vi "WriteOctToFile.vi"(8 "Error In":errorcluster, 9 "Scan.lvclass":refnum<class "Scan.lvclass">, 10 "Refnum in":refnum<file>, 11 "Queue in":refnum<queue>) -> (0 "error out":errorcluster, 1 "refnum out":refnum<file>, 2 "Frame number":dbl, 3 "prepend array or string size? (T)":bool)   [LabVIEW 2017]
uses:
  classes/Scans/Scan.lvclass
  classes/Scans/Scan.lvclass/Scan.ctl
  classes/Scans/Read B scans.vi
  classes/Scans/Read Repeat B scans.vi
  classes/Scans/Read C scans.vi
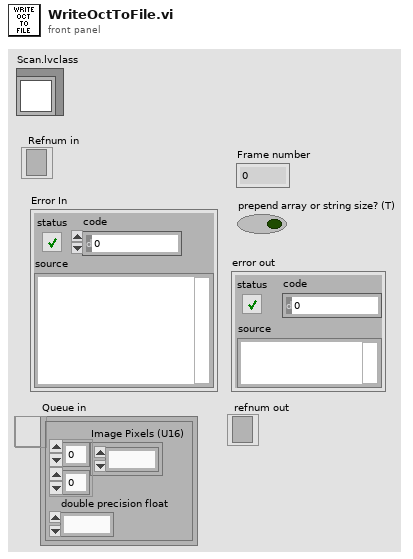
[diagram p1: front panel]
types:
  T1 = enum16{"big-endian, network order", "native, host order", "little-endian"}
  T2 = cluster{"Image Pixels (U16)":u16[][], "double precision float":dbl}
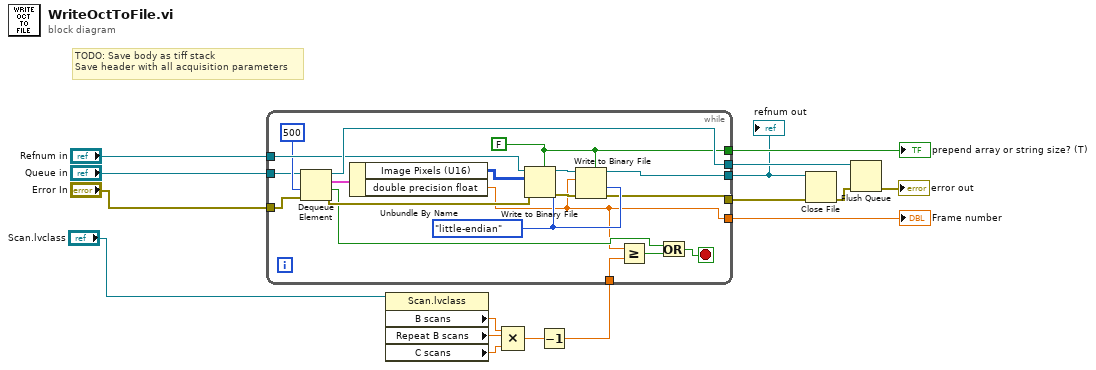
[diagram p0: block diagram]
diagram:
  # "TODO: Save body as tiff stack\nSave header with all acquisition parameters"
  n1 = property class="Scan.lvclass"(reference="Scan.lvclass") -> ("B scans"=w5:dbl, "Repeat B scans"=w4:dbl, "C scans"=w3:dbl)  [unwired: 1 in, 2 out]
  n2 = Compound Arithmetic op=MULTIPLY(w5, w4, w3) -> (w2:dbl)
  n3 = Decrement(x=w2) -> (x-1=w1:dbl)
  n4 = while {
    tunnel: "Queue in" -> [w18]
    tunnel: "Error In" -> [w17]
    tunnel: "Refnum in" -> [w29]
    tunnel: [w26] -> w13
    tunnel: [w34] -> w16
    tunnel: w1 -> [w33]
    tunnel: [w23] -> w12
    tunnel: [w22] -> w11
    tunnel: [w19] -> w7
    stop <- w20 stop-if-true
    w27 = T1."little-endian" ("byte order (0:big-endian, network order)")
    w26 = FALSE ("prepend array or string size? (T)")
    n5 = Dequeue Element(queue=w18, timeout in ms (-1)=500, error in (no error)=w17) -> (queue out=w34:refnum<queue>, element=w25:T2, timed out?=w31:bool, error out=w35:errorcluster)
    n6 = Unbundle By Name(w25) -> ("Image Pixels (U16)"=w24:u16[][], "double precision float"=w19:dbl)
    n7 = Write to Binary File(file (use dialog)=w29, data=w24, error in=w35, 5:w26, 9:w27) -> (refnum out=w28:refnum<file>, error out=w30:errorcluster)  [unwired: 1 in, 1 out]
    n8 = Write to Binary File(file (use dialog)=w28, data=w19, error in=w30, 5:w26, 9:w27) -> (refnum out=w22:refnum<file>, error out=w23:errorcluster)  [unwired: 1 in, 1 out]
    n9 = Greater Or Equal?(x=w19, y=w33) -> (x >= y?=w32:bool)
    n10 = Or(x=w31, y=w32) -> (x .or. y?=w20:bool)
  }
  "prepend array or string size? (T)" <- w13
  "Frame number" <- w7
  "refnum out" <- w11
  n11 = Close File(refnum=w11, error in=w12) -> (error out=w14:errorcluster)  [unwired: 1 out]
  n12 = Flush Queue(queue=w16, error in (no error)=w14) -> (error out=→"error out":errorcluster)  [unwired: 2 out]
